vi "LINXseñal cuadrada.vi"() -> ()   [LabVIEW 2023]
doc: "This example demonstrates how to read one channel of digital input from a LINX device."
uses:
  <vilib>/MakerHub/LINX/Public/Peripherals/Digital/Digital Write 1 Chan.vi
  <vilib>/MakerHub/LINX/Public/Peripherals/Digital/Digital Write N Chans.vi
  <vilib>/MakerHub/LINX/Private/Local IO/LinxDigitalWrite.vi
  <vilib>/MakerHub/LINX/Public/Utilities/Check Channel.vi
  <vilib>/MakerHub/LINX/Public/Utilities/Open Serial.vi
  <vilib>/MakerHub/LINX/Private/Utilties/Generate Error.vi
  <vilib>/MakerHub/LINX/LMH-LINX.lvlib
panel:
  in  "Stop Button 2":bool
  in  "Frecuencia":dbl
  in  "Canal Digital":u8=2
  in  "Stop Button":bool
  in  "Puerto Serie":refnum<visa-resource-name>
  # "Ajustes de Software"
  # "Ajustes de microcontrolador"
  # "Señal Cudrada:"
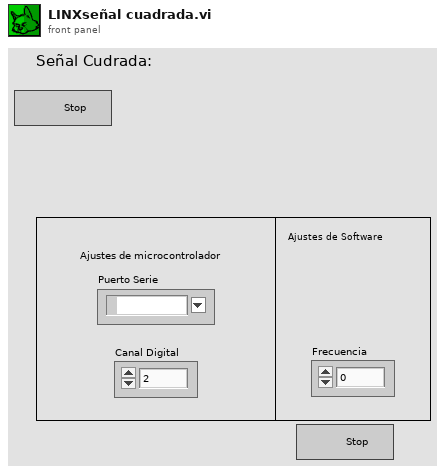
[diagram p1: front panel]
types:
  T1 = typedef "LMH-LINX.lvlib/LINX Ref.ctl" = cluster{"IO":T2, "Interface":T3, "LINX Device Config":T4}
  T2 = typedef "LMH-LINX.lvlib/Platform.ctl" = enum16{"Remote", "Local"}
  T3 = typedef "LMH-LINX.lvlib/Interface.ctl" = enum16{"Serial", "TCP"}
  T4 = typedef "LMH-LINX.lvlib/Device.lvlib/LINX Device Config.ctl" = cluster{"Interface":T3, "COM Port":refnum<visa-resource-name>, "TCP Configuration":T5, "Device Family":u8, "Device ID":u8, "Device Name":string, "TCP Ref":refnum<k5>, "Channels":T6}
  T5 = typedef "LMH-LINX.lvlib/Device.lvlib/TCP Config.ctl" = cluster{"IP Address":string, "Port":u16}
  T6 = typedef "LMH-LINX.lvlib/Channels.ctl" = cluster{"DI":u8[], "DO":u8[], "AI":u8[], "AO":u8[], "PWM":u8[], "QE":u8[], "UART":u8[], "I2C 2":u8[], "SPI":u8[], "CAN":u8[], "Servo":u8[], "AI Ref (V)":dbl, "AI Resolution (Bits)":u8, "AO Ref (V)":dbl, "AO Resolution (Bits)":u8}
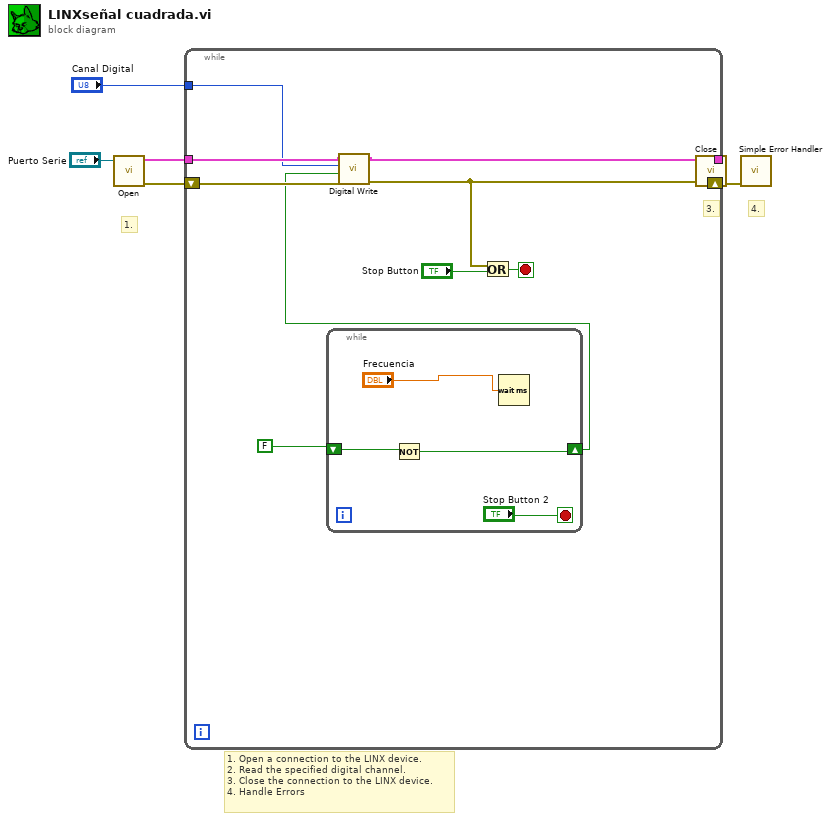
[diagram p0: block diagram]
diagram:
  # "1. Open a connection to the LINX device.\n2. Read the specified digital channel.\n3. Close the connection to the LINX device.\n4. Handle Errors"
  # "4."
  # "3."
  # "1."
  n1 = call-poly <vilib>:"Open.vi"("Serial Port"="Puerto Serie") -> ("Error Out"=w6:errorcluster, "LINX Resource"=w7:T1)  [unwired: 8 in, 1 out]
  n2 = while {
    tunnel: w7 -> [w12]
    tunnel: [w13] -> w5
    shift-right: [w14] -> w4
    shift-left: w6 -> [w11]
    tunnel: "Canal Digital" -> [w10]
    stop <- w16 stop-if-true
    n3 = while {
      shift-right: [w17] -> w8
      shift-left: FALSE -> [w18]
      stop <- "Stop Button 2" stop-if-true
      n4 = Not(x=w18) -> (.not. x?=w17:bool)
      n5 = Wait (ms)(milliseconds to wait="Frecuencia") -> ()  [unwired: 1 out]
    }
    n6 = call-poly <vilib>:"Digital Write.vi"("Error In"=w11, "Output Value"=w8, "DO Channel"=w10, "LINX Resource"=w12) -> ("Error Out"=w14:errorcluster, "LINX Resource"=w13:T1)  [unwired: 6 in]
    n7 = Or(x=w14, y="Stop Button") -> (x .or. y?=w16:bool)
  }
  n8 = call <vilib>:"Close.vi"("Error In"=w4, "LINX Resource"=w5) -> ("Error Out"=w2:errorcluster)  [unwired: 9 in]
  n9 = call <vilib>:"Simple Error Handler.vi"("error in (no error)"=w2) -> ()  [unwired: 4 in, 5 out]
